vi "log analysis_gps.vi"() -> ()   [LabVIEW 2019] (continued)
178.674099\t119.545505\t7.850800\t-0.685777\t0.071314\t-179.533156\t0.281000\t0.057000\n\t\n15:42:58.0\tlog_raw\tgps_raw\t\tsystem status\tnormal 2 27.600000 0 0\trobot status\t178.530847\t119.555487\t7.852900\t-0.681543\t0.074991\t-178.454031\t0.250000\t0.099000\n\t\n15:42:58.5\tlog_raw\tgps_raw\t\tsystem status\tnormal 2 27.700000 0 0\trobot status\t178.388527\t119.563164\t7.854800\t-0.589771\t-0.039623\t-177.691683\t0.355000\t-0.076000\n\t\n15:42:59.0\tlog_raw\tgps_raw\t#INSPVAXA,USB3,0,48.0,FINESTEERING,2107,283397.000,02008000,471d,15824;INS_ALIGNMENT_COMPLETE,INS_RTKFIXED,37.37120756158,126.72284723555,7.8555,22.3000,0.0154,-0.2918,-0.0108,-0.634674297,-0.085063668,267.337636421,0.4417,0.2975,0.5723,0.1133,0.0929,0.0782,0.0967,0.1016,4.9878,0f000001,0*8fe1902c\n\tsystem status\tnormal 2 27.800000 0 0\trobot status\t178.231220\t119.569034\t7.855500\t-0.634674\t-0.085064\t-177.337636\t0.230000\t0.096000\n\t\n15:42:59.5\tlog_raw\tgps_raw\t\tsystem status\tnormal 2 27.900000 0 0\trobot status\t178.104677\t119.573703\t7.856600\t-0.691004\t0.066213\t-177.257686\t0.292000\t-0.004000\n\t\n15:43:00.0\tlog_raw\tgps_raw\t\tsystem status\tnormal 2 27.800000 0 0\trobot status\t178.014430\t119.582125\t7.857700\t-0.560476\t0.164777\t-177.081673\t0.289000\t-0.046000\n\t\n15:43:00.5\tlog_raw\tgps_raw\t#INSPVAXA,USB3,0,46.0,FINESTEERING,2107,283398.500,02000000,471d,15824;INS_ALIGNMENT_COMPLETE,INS_RTKFIXED,37.37120769045,126.72284269521,7.8578,22.3000,0.0082,-0.2767,-0.0005,-0.866355787,-0.085585905,267.490403578,0.4423,0.2980,0.5726,0.1137,0.0929,0.0782,0.0966,0.1016,4.9900,0f000001,0*ee0dcbd5\n\tsystem status\tnormal 2 27.900000 0 0\trobot status\t177.829044\t119.583345\t7.857800\t-0.866356\t-0.085586\t-177.490404\t0.291000\t-0.016000\n\t\n15:43:01.0\tlog_raw\tgps_raw\t#INSPVAXA,USB3,0,46.0,FINESTEERING,2107,283399.000,02000000,471d,15824;INS_ALIGNMENT_COMPLETE,INS_RTKFIXED,37.37120774226,126.72284145946,7.8578,22.3000,0.0199,-0.3107,0.0000,-0.861107937,-0.016080151,267.485200406,0.4423,0.2980,0.5726,0.1137,0.0929,0.0782,0.0966,0.1016,4.9900,0f000001,0*0e2ee5eb\n\tsystem status\tnormal 2 27.900000 0 0\trobot status\t177.719583\t119.589098\t7.857800\t-0.861108\t-0.016080\t-177.485200\t0.296000\t-0.009000\n\t\n15:43:01.5\tlog_raw\tgps_raw\t\tsystem status\tnormal 2 27.900000 0 0\trobot status\t177.583399\t119.592846\t7.858100\t-0.914716\t-0.066763\t-177.678459\t0.294000\t-0.080000\n\t\n15:43:02.0\tlog_raw\tgps_raw\t\tsystem status\tnormal 2 27.900000 0 0\trobot status\t177.430654\t119.597965\t7.857300\t-1.000637\t-0.107557\t-178.105388\t0.316000\t-0.089000\n\t\n15:43:02.5\tlog_raw\tgps_raw\t#INSPVAXA,USB3,0,49.0,FINESTEERING,2107,283400.500,02008000,471d,15824;INS_ALIGNMENT_COMPLETE,INS_RTKFIXED,37.37120790493,126.72283644279,7.8568,22.3000,0.0415,-0.3200,-0.0102,-0.992860449,-0.204263174,269.501464610,0.4444,0.2986,0.5733,0.1141,0.0930,0.0783,0.0966,0.1016,4.9910,0f000001,0*94df5475\n\tsystem status\tnormal 2 27.600000 0 0\trobot status\t177.275215\t119.607161\t7.856800\t-0.992860\t-0.204263\t-179.501465\t0.300000\t-0.089000\n\t\n15:43:03.0\tlog_raw\tgps_raw\t\tsystem status\tnormal 2 27.400000 0 0\trobot status\t177.149847\t119.619751\t7.856100\t-1.032172\t-0.114714\t178.589566\t0.300000\t-0.076000\n\t\n15:43:03.5\tlog_raw\tgps_raw\t#INSPVAXA,USB3,0,51.0,FINESTEERING,2107,283401.500,02008000,471d,15824;INS_ALIGNMENT_COMPLETE,INS_RTKFIXED,37.37120822785,126.72283327218,7.8567,22.3000,0.0378,-0.2848,0.0013,-0.896017543,0.041472970,274.456577076,0.4448,0.2985,0.5735,0.1139,0.0930,0.0783,0.0966,0.1016,4.9907,0f000001,0*a1fc700f\n\tsystem status\tnormal 2 27.300000 4 0\trobot status\t177.008302\t119.641208\t7.856600\t-0.892681\t-0.081437\t175.816173\t0.307000\t-0.101000\n\t\n15:43:04.0\tlog_raw\tgps_raw\t#INSPVAXA,USB3,0,51.0,FINESTEERING,2107,283402.000,02008000,471d,15824;INS_ALIGNMENT_COMPLETE,INS_RTKFIXED,37.37120847864,126.72283165681,7.8567,22.3000,0.0753,-0.3061,0.0004,-0.849514538,-0.111394273,277.112069112,0.4448,0.2985,0.5735,0.1139,0.0930,0.0783,0.0966,0.1016,4.9907,0f000001,0*e592cbf0\n\tsystem status\tnormal 2 27.200000 4 0\trobot status\t176.851281\t119.670843\t7.856700\t-0.849515\t-0.111394\t172.887931\t0.290000\t-0.092000\n\t\n15:43:04.5\tlog_raw\tgps_raw\t#INSPVAXA,USB3,0,40.0,FINESTEERING,2107,283402.500,02008000,471d,15824;INS_ALIGNMENT_COMPLETE,INS_RTKFIXED,37.37120871914,126.72283047198,7.8552,22.3000,0.0392,-0.0732,-0.0063,-0.879415981,-0.139080353,278.991486756,0.4452,0.2985,0.5736,0.1139,0.0932,0.0783,0.0967,0.1016,4.9892,0f000001,0*49d1c048\n\tsystem status\tnormal 2 27.500000 0 0\trobot status\t176.746330\t119.697537\t7.855200\t-0.879416\t-0.139080\t171.008513\t0.083000\t-0.016000\n\t\n15:43:05.0\tlog_raw\tgps_raw\t#INSPVAXA,USB3,0,40.0,FINESTEERING,2107,283403.000,02008000,471d,15824;INS_ALIGNMENT_COMPLETE,INS_RTKFIXED,37.37120908297,126.72282892192,7.8525,22.3000,0.0902,-0.2460,-0.0094,-0.757562601,-0.250041594,280.800208389,0.4452,0.2985,0.5736,0.1139,0.0932,0.0783,0.0967,0.1016,4.9892,0f000001,0*49bd1315\n\tsystem status\tnormal 2 27.600000 0 0\trobot status\t176.609029\t119.737920\t7.852500\t-0.757563\t-0.250042\t169.199792\t0.253000\t-0.048000\n\t\n15:43:05.5\tlog_raw\tgps_raw\t#INSPVAXA,USB3,0,49.5,FINESTEERING,2107,283403.500,02008000,471d,15824;INS_ALIGNMENT_COMPLETE,INS_RTKFIXED,37.37120946303,126.72282732667,7.8498,22.3000,0.0944,-0.2806,-0.0193,-0.668842152,-0.504747549,282.253589377,0.4448,0.2984,0.5737,0.1136,0.0933,0.0783,0.0967,0.1016,4.9866,0f000001,0*5936c3a3\n\tsystem status\tnormal 2 27.600000 0 0\trobot status\t176.467724\t119.780103\t7.849800\t-0.668842\t-0.504748\t167.746411\t0.286000\t-0.039000\n\t\n15:43:06.0\tlog_raw\tgps_raw\t\tsystem status\tnormal 2 27.700000 0 0\trobot status\t176.338393\t119.821680\t7.846400\t-0.619203\t-0.637590\t166.743344\t0.300000\t-0.021000\n\t\n15:43:06.5\tlog_raw\tgps_raw\t#INSPVAXA,USB3,0,44.5,FINESTEERING,2107,283404.500,02000000,471d,15824;INS_ALIGNMENT_COMPLETE,INS_RTKFIXED,37.37121031708,126.72282412618,7.8426,22.3000,0.0922,-0.2745,-0.0175,-0.508504474,-0.605332941,283.953665433,0.4448,0.2984,0.5737,0.1137,0.0932,0.0783,0.0967,0.1016,4.9838,0f000001,0*f5451d9e\n\tsystem status\tnormal 2 27.800000 0 0\trobot status\t176.184230\t119.874896\t7.842600\t-0.508504\t-0.605333\t166.046335\t0.306000\t0.002000\n\t\n15:43:07.0\tlog_raw\tgps_raw\t\tsystem status\tnormal 2 27.800000 0 0\trobot status\t176.058492\t119.920630\t7.837600\t-0.353083\t-0.545601\t165.722125\t0.254000\t-0.062000\n\t\n15:43:07.5\tlog_raw\tgps_raw\t#INSPVAXA,USB3,0,43.5,FINESTEERING,2107,283405.500,02000000,471d,15824;INS_ALIGNMENT_COMPLETE,INS_RTKFIXED,37.37121122876,126.72282101701,7.8318,22.3000,0.1002,-0.2755,-0.0247,-0.139047561,-0.305791959,284.480251115,0.4442,0.2983,0.5736,0.1136,0.0932,0.0782,0.0967,0.1016,4.9810,0f000001,0*98e81a7f\n\tsystem status\tnormal 2 27.900000 0 0\trobot status\t175.908825\t119.976084\t7.831800\t-0.139048\t-0.305792\t165.519749\t0.289000\t-0.013000\n\t\n15:43:08.0\tlog_raw\tgps_raw\t#INSPVAXA,USB3,0,43.5,FINESTEERING,2107,283406.000,02000000,471d,15824;INS_ALIGNMENT_COMPLETE,INS_RTKFIXED,37.37121169397,126.72281951047,7.8268,22.3000,0.1108,-0.2868,-0.0208,0.099651120,-0.291418852,284.605342241,0.4442,0.2983,0.5736,0.1136,0.0932,0.0782,0.0967,0.1016,4.9810,0f000001,0*55374de0\n\tsystem status\tnormal 2 27.900000 0 0\trobot status\t175.775378\t120.027718\t7.826800\t0.099651\t-0.291419\t165.394658\t0.302000\t0.023000\n\t\n15:43:08.5\tlog_raw\tgps_raw\t#INSPVAXA,USB3,0,49.5,FINESTEERING,2107,283406.500,02000000,471d,15824;INS_ALIGNMENT_COMPLETE,INS_RTKFIXED,37.37121212971,126.72281808061,7.8238,22.3000,0.1054,-0.2584,-0.0109,0.137601109,-0.336757445,284.673154927,0.4438,0.2982,0.5735,0.1136,0.0935,0.0782,0.0967,0.1016,4.9790,0f000001,0*e60377c5\n\tsystem status\tnormal 2 27.900000 0 0\trobot status\t175.648723\t120.076081\t7.823800\t0.137601\t-0.336757\t165.326845\t0.291000\t0.030000\n\t\n15:43:09.0\tlog_raw\tgps_raw\t#INSPVAXA,USB3,0,49.5,FINESTEERING,2107,283407.000,02000000,471d,15824;INS_ALIGNMENT_COMPLETE,INS_RTKFIXED,37.37121262713,126.72281640166,7.8194,22.3000,0.1069,-0.3011,-0.0264,0.109820957,-0.453228449,284.767303943,0.4438,0.2982,0.5735,0.1136,0.0935,0.0782,0.0967,0.1016,4.9790,0f000001,0*3f427643\n\tsystem status\tnormal 2 27.900000 0 0\trobot status\t175.500005\t120.131290\t7.819400\t0.109821\t-0.453228\t165.232696\t0.243000\t0.059000\n\t\n15:43:09.5\tlog_raw\tgps_raw\t#INSPVAXA,USB3,0,48.0,FINESTEERING,2107,283407.500,02000000,471d,15824;INS_ALIGNMENT_COMPLETE,INS_RTKFIXED,37.37121306195,126.72281499649,7.8146,22.3000,0.1240,-0.3347,-0.0132,0.207501666,-0.436324558,284.580204536,0.4442,0.2982,0.5735,0.1137,0.0934,0.0782,0.0967,0.1017,4.9771,0f000001,0*8c70faff\n\tsystem status\tnormal 2 27.800000 0 0\trobot status\t175.375537\t120.179551\t7.814600\t0.207502\t-0.436325\t165.419795\t0.329000\t0.008000\n\t\n15:43:10.0\tlog_raw\tgps_raw\t#INSPVAXA,USB3,0,48.0,FINESTEERING,2107,283408.000,02000000,471d,15824;INS_ALIGNMENT_COMPLETE,INS_RTKFIXED,37.37121354821,126.72281341269,7.8101,22.3000,0.1116,-0.3074,-0.0226,0.525843943,-0.411708262,284.163389107,0.4442,0.2982,0.5735,0.1137,0.0934,0.0782,0.0967,0.1017,4.9771,0f000001,0*c1d0c0d0\n\tsystem status\tnormal 2 27.800000 0 0\trobot status\t175.235246\t120.233521\t7.810100\t0.525844\t-0.411708\t165.836611\t0.230000\t0.127000\n\t\n15:43:10.5\tlog_raw\tgps_raw\t#INSPVAXA,USB3,0,44.0,FINESTEERING,2107,283408.500,02000000,471d,15824;INS_ALIGNMENT_COMPLETE,INS_RTKFIXED,37.37121398943,126.72281189680,7.8055,22.3000,0.1138,-0.2746,-0.0275,0.675393790,-0.337920064,283.271814178,0.4441,0.2981,0.5734,0.1138,0.0936,0.0782,0.0967,0.1017,4.9759,0f000001,0*ad4dbf0b\n\tsystem status\tnormal 2 27.700000 0 0\trobot status\t175.100971\t120.282493\t7.805500\t0.675394\t-0.337920\t166.728186\t0.325000\t-0.019000\n\t\n15:43:11.0\tlog_raw\tgps_raw\t#INSPVAXA,USB3,0,44.0,FINESTEERING,2107,283409.000,02000000,471d,15824;INS_ALIGNMENT_COMPLETE,INS_RTKFIXED,37.37121442754,126.72281035382,7.7998,22.3000,0.1067,-0.2915,-0.0280,0.822552391,-0.280575690,282.018938014,0.4441,0.2981,0.5734,0.1138,0.0936,0.0782,0.0967,0.1017,4.9759,0f000001,0*67fc65b3\n\tsystem status\tnormal 2 27.500000 0 0\trobot status\t174.964297\t120.331119\t7.799800\t0.822552\t-0.280576\t167.981062\t0.275000\t0.073000\n\t\n15:43:11.5\tlog_raw\tgps_raw\t#INSPVAXA,USB3,0,49.0,FINESTEERING,2107,283409.500,02000000,471d,15824;INS_ALIGNMENT_COMPLETE,INS_RTKFIXED,37.37121478666,126.72280882264,7.7967,22.3000,0.1036,-0.2896,-0.0167,0.817605955,-0.233379824,280.341751622,0.4442,0.2981,0.5733,0.1139,0.0934,0.0782,0.0968,0.1017,4.9750,0f000001,0*d948c100\n\tsystem status\tnormal 2 27.300000 0 0\trobot status\t174.828667\t120.370979\t7.796700\t0.817606\t-0.233380\t169.658248\t0.311000\t0.063000\n\t\n15:43:12.0\tlog_raw\tgps_raw\t#INSPVAXA,USB3,0,49.0,FINESTEERING,2107,283410.000,02000000,471d,15824;INS_ALIGNMENT_COMPLETE,INS_RTKFIXED,37.37121511578,126.72280728000,7.7945,22.3000,0.0801,-0.2984,-0.0279,0.678250969,-0.053144715,278.846138365,0.4442,0.2981,0.5733,0.1139,0.0934,0.0782,0.0968,0.1017,4.9750,0f000001,0*ea5c4675\n\tsystem status\tnormal 2 27.400000 0 0\trobot status\t174.692023\t120.407509\t7.794500\t0.678251\t-0.053145\t171.153862\t0.300000\t0.053000\n\t\n15:43:12.5\tlog_raw\tgps_raw\t#INSPVAXA,USB3,0,50.0,FINESTEERING,2107,283410.500,02000000,471d,15824;INS_ALIGNMENT_COMPLETE,INS_RTKFIXED,37.37121543638,126.72280574107,7.7946,22.3000,0.0881,-0.2945,-0.0308,0.799531851,-0.090684476,277.306863329,0.4440,0.2981,0.5734,0.1139,0.0931,0.0782,0.0968,0.1016,4.9749,0f000001,0*8afda85b\n\tsystem status\tnormal 2 27.400000 0 0\trobot status\t174.555707\t120.443093\t7.794600\t0.799532\t-0.090684\t172.693137\t0.303000\t0.051000\n\t\n15:43:13.0\tlog_raw\tgps_raw\t#INSPVAXA,USB3,0,50.0,FINESTEERING,2107,283411.000,02000000,471d,15824;INS_ALIGNMENT_COMPLETE,INS_RTKFIXED,37.37121573081,126.72280419949,7.7932,22.3000,0.0856,-0.2853,-0.0213,0.874963838,0.088876900,275.787048290,0.4440,0.2981,0.5734,0.1139,0.0931,0.0782,0.0968,0.1016,4.9749,0f000001,0*8eff61ca\n\tsystem status\tnormal 2 27.400000 0 0\trobot status\t174.419156\t120.475773\t7.793200\t0.874964\t0.088877\t174.212952\t0.295000\t0.043000\n\t\n15:43:13.5\tlog_raw\tgps_raw\t#INSPVAXA,USB3,0,47.0,FINESTEERING,2107,283411.500,02000000,471d,15824;INS_ALIGNMENT_COMPLETE,INS_RTKFIXED,37.37121596120,126.72280262366,7.7899,22.3000,0.0704,-0.2845,-0.0255,0.751254674,0.247689552,274.576260626,0.4438,0.2979,0.5732,0.1139,0.0930,0.0782,0.0968,0.1016,4.9755,0f000001,0*e84a82b6\n\tsystem status\tnormal 2 27.600000 0 0\trobot status\t174.279572\t120.501346\t7.789900\t0.751255\t0.247690\t175.423739\t0.301000\t0.040000\n\t\n15:43:14.0\tlog_raw\tgps_raw\t#INSPVAXA,USB3,0,47.0,FINESTEERING,2107,283412.000,02000000,471d,15824;INS_ALIGNMENT_COMPLETE,INS_RTKFIXED,37.37121617740,126.72280126848,7.7873,22.3000,0.0873,-0.4025,-0.0234,0.616180414,0.315751061,274.011690427,0.4438,0.2979,0.5732,0.1139,0.0930,0.0782,0.0968,0.1016,4.9755,0f000001,0*aa33c281\n\tsystem status\tnormal 2 27.600000 0 0\trobot status\t174.159532\t120.525343\t7.787300\t0.616180\t0.315751\t175.988310\t0.464000\t-0.135000\n\t\n15:43:14.5\tlog_raw\tgps_raw\t#INSPVAXA,USB3,0,49.0,FINESTEERING,2107,283412.500,02000000,471d,15824;INS_ALIGNMENT_COMPLETE,INS_RTKFIXED,37.37121638911,126.72279968745,7.7862,22.3000,0.0846,-0.3281,-0.0274,0.679733503,0.333649216,273.348704844,0.4441,0.2978,0.5733,0.1135,0.0929,0.0782,0.0967,0.1016,4.9761,0f000001,0*b2c3b0d0\n\tsystem status\tnormal 2 27.700000 0 0\trobot status\t174.019487\t120.548843\t7.786200\t0.679734\t0.333649\t176.651295\t0.285000\t0.061000\n\t\n15:43:15.0\tlog_raw\tgps_raw\t#INSPVAXA,USB3,0,49.0,FINESTEERING,2107,283413.000,02000000,471d,15824;INS_ALIGNMENT_COMPLETE,INS_RTKFIXED,37.37121660586,126.72279809431,7.7843,22.3000,0.0703,-0.2977,-0.0214,0.740409973,0.249491929,272.781944471,0.4441,0.2978,0.5733,0.1135,0.0929,0.0782,0.0967,0.1016,4.9761,0f000001,0*f60b4ece\n\tsystem status\tnormal 2 27.700000 0 0\trobot status\t173.878369\t120.572902\t7.784300\t0.740410\t0.249492\t177.218056\t0.285000\t0.039000\n\t\n15:43:15.5\tlog_raw\tgps_raw\t#INSPVAXA,USB3,0,52.0,FINESTEERING,2107,283413.500,02000000,471d,15824;INS_ALIGNMENT_COMPLETE,INS_RTKFIXED,37.37121678011,126.72279647899,7.7842,22.3000,0.0611,-0.2896,-0.0156,0.541768048,0.276425000,272.440789392,0.4443,0.2978,0.5734,0.1137,0.0930,0.0783,0.0967,0.1016,4.9772,0f000001,0*dee707a2\n\tsystem status\tnormal 2 27.800000 0 0\trobot status\t173.735287\t120.592244\t7.784200\t0.541768\t0.276425\t177.559211\t0.303000\t0.023000\n\t\n15:43:16.0\tlog_raw\tgps_raw\t#INSPVAXA,USB3,0,52.0,FINESTEERING,2107,283414.000,02000000,471d,15824;INS_ALIGNMENT_COMPLETE,INS_RTKFIXED,37.37121695844,126.72279487453,7.7833,22.3000,0.0562,-0.2987,-0.0221,0.305746211,0.346254228,272.319331007,0.4443,0.2978,0.5734,0.1137,0.0930,0.0783,0.0967,0.1016,4.9772,0f000001,0*5e10dc17\n\tsystem status\tnormal 2 27.800000 0 0\trobot status\t173.593167\t120.612039\t7.783300\t0.305746\t0.346254\t177.680669\t0.255000\t0.072000\n\t\n15:43:16.5\tlog_raw\tgps_raw\t#INSPVAXA,USB3,0,50.0,FINESTEERING,2107,283414.500,02000000,471d,15824;INS_ALIGNMENT_COMPLETE,INS_RTKFIXED,37.37121711379,126.72279330042,7.7828,22.3000,0.0616,-0.3002,-0.0329,0.276756604,0.384134091,272.213822291,0.4446,0.2977,0.5735,0.1137,0.0931,0.0783,0.0967,0.1016,4.9781,0f000001,0*58d30e64\n\tsystem status\tnormal 2 27.800000 0 0\trobot status\t173.453735\t120.629283\t7.782800\t0.276757\t0.384134\t177.786178\t0.325000\t-0.049000\n\t\n15:43:17.0\tlog_raw\tgps_raw\t#INSPVAXA,USB3,0,50.0,FINESTEERING,2107,283415.000,02000000,471d,15824;INS_ALIGNMENT_COMPLETE,INS_RTKFIXED,37.37121729157,126.72279172002,7.7811,22.3000,0.0636,-0.2842,-0.0222,0.415011946,0.501817180,272.226800833,0.4446,0.2977,0.5735,0.1137,0.0931,0.0783,0.0967,0.1016,4.9781,0f000001,0*6d269faa\n\tsystem status\tnormal 2 27.900000 0 0\trobot status\t173.313745\t120.649017\t7.781100\t0.415012\t0.501817\t177.773199\t0.252000\t0.068000\n\t\n15:43:17.5\tlog_raw\tgps_raw\t#INSPVAXA,USB3,0,47.5,FINESTEERING,2107,283415.500,02000000,471d,15824;INS_ALIGNMENT_COMPLETE,INS_RTKFIXED,37.37121745091,126.72279017522,7.7808,22.3000,0.0665,-0.2955,-0.0219,0.380400509,0.552941969,272.302095056,0.4463,0.2979,0.5741,0.1141,0.0931,0.0783,0.0967,0.1016,4.9784,0f000001,0*a1df6ecd\n\tsystem status\tnormal 2 27.900000 0 0\trobot status\t173.176909\t120.666704\t7.780800\t0.380401\t0.552942\t177.697905\t0.302000\t-0.016000\n\t\n15:43:18.0\tlog_raw\tgps_raw\t#INSPVAXA,USB3,0,47.5,FINESTEERING,2107,283416.000,02000000,471d,15824;INS_ALIGNMENT_COMPLETE,INS_RTKFIXED,37.37121761561,126.72278863452,7.7803,22.3000,0.0694,-0.2870,-0.0195,0.176632637,0.631844769,272.368772552,0.4463,0.2979,0.5741,0.1141,0.0931,0.0783,0.0967,0.1016,4.9784,0f000001,0*101cc811\n\tsystem status\tnormal 2 27.900000 0 0\trobot status\t173.040437\t120.684986\t7.780300\t0.176633\t0.631845\t177.631227\t0.294000\t-0.025000\n\t\n15:43:18.5\tlog_raw\tgps_raw\t#INSPVAXA,USB3,0,48.5,FINESTEERING,2107,283416.500,02000000,471d,15824;INS_ALIGNMENT_COMPLETE,INS_RTKFIXED,37.37121775832,126.72278713599,7.7826,22.3000,0.0697,-0.2192,-0.0178,0.097264946,0.637535268,272.514997324,0.4476,0.2980,0.5744,0.1141,0.0933,0.0783,0.0967,0.1016,4.9780,0f000001,0*de8fa7bd\n\tsystem status\tnormal 2 27.900000 0 0\trobot status\t172.907699\t120.700827\t7.782600\t0.097265\t0.637535\t177.485003\t0.270000\t-0.019000\n\t\n15:43:19.0\tlog_raw\tgps_raw\t#INSPVAXA,USB3,0,48.5,FINESTEERING,2107,283417.000,02000000,471d,15824;INS_ALIGNMENT_COMPLETE,INS_RTKFIXED,37.37121791673,126.72278556304,7.7837,22.3000,0.0663,-0.3100,-0.0205,0.059332705,0.713618061,272.644367778,0.4476,0.2980,0.5744,0.1141,0.0933,0.0783,0.0967,0.1016,4.9780,0f000001,0*0eada2f0\n\tsystem status\tnormal 2 27.900000 0 0\trobot status\t172.768370\t120.718411\t7.783700\t0.059333\t0.713618\t177.355632\t0.311000\t-0.019000\n\t\n15:43:19.5\tlog_raw\tgps_raw\t#INSPVAXA,USB3,0,49.5,FINESTEERING,2107,283417.500,02000000,471d,15824;INS_ALIGNMENT_COMPLETE,INS_RTKFIXED,37.37121805927,126.72278401761,7.7854,22.3000,0.0733,-0.3034,-0.0199,-0.089736281,0.682506792,272.907308438,0.4484,0.2980,0.5747,0.1140,0.0932,0.0783,0.0967,0.1016,4.9768,0f000001,0*d6901b99\n\tsystem status\tnormal 2 27.900000 0 0\trobot status\t172.631478\t120.734234\t7.785400\t-0.089736\t0.682507\t177.092692\t0.296000\t-0.026000\n\t\n15:43:20.0\tlog_raw\tgps_raw\t#INSPVAXA,USB3,0,49.5,FINESTEERING,2107,283418.000,02000000,471d,15824;INS_ALIGNMENT_COMPLETE,INS_RTKFIXED,37.37121822786,126.72278229435,7.7864,22.3000,0.0757,-0.2957,-0.0211,-0.132925530,0.544261576,273.127275115,0.4484,0.2980,0.5747,0.1140,0.0932,0.0783,0.0967,0.1016,4.9768,0f000001,0*048d27a0\n\tsystem status\tnormal 2 27.900000 0 0\trobot status\t172.478835\t120.752948\t7.786400\t-0.132926\t0.544262\t176.872725\t0.297000\t-0.022000\n\t\n15:43:20.5\tlog_raw\tgps_raw\t#INSPVAXA,USB3,0,48.5,FINESTEERING,2107,283418.500,02000000,471d,15824;INS_ALIGNMENT_COMPLETE,INS_RTKFIXED,37.37121838802,126.72278063938,7.7901,22.3000,0.0744,-0.3140,-0.0189,-0.074171217,0.383892357,273.451467378,0.4479,0.2973,0.5742,0.1138,0.0931,0.0783,0.0966,0.1015,4.9755,0f000001,0*a7f0c313\n\tsystem status\tnormal 2 27.900000 0 0\trobot status\t172.332240\t120.770726\t7.790100\t-0.074171\t0.383892\t176.548533\t0.318000\t-0.017000\n\t\n15:43:21.0\tlog_raw\tgps_raw\t#INSPVAXA,USB3,0,48.5,FINESTEERING,2107,283419.000,02000000,471d,15824;INS_ALIGNMENT_COMPLETE,INS_RTKFIXED,37.37121856246,126.72277896327,7.7932,22.3000,0.0727,-0.3040,-0.0212,-0.024906260,0.224477115,273.793356519,0.4479,0.2973,0.5742,0.1138,0.0931,0.0783,0.0966,0.1015,4.9755,0f000001,0*a3bde9c9\n\tsystem status\tnormal 2 27.900000 0 0\trobot status\t172.183773\t120.790089\t7.793200\t-0.024906\t0.224477\t176.206643\t0.309000\t-0.022000\n\t\n15:43:21.5\tlog_raw\tgps_raw\t#INSPVAXA,USB3,0,48.5,FINESTEERING,2107,283419.500,02000000,471d,15824;INS_ALIGNMENT_COMPLETE,INS_RTKFIXED,37.37121873521,126.72277734418,7.7960,22.3000,0.0758,-0.3154,-0.0078,-0.021214683,0.148956013,274.268869002,0.4473,0.2969,0.5737,0.1137,0.0929,0.0783,0.0966,0.1015,4.9747,0f000001,0*df94383f\n\tsystem status\tnormal 2 27.800000 0 0\trobot status\t172.040357\t120.809265\t7.796000\t-0.021215\t0.148956\t175.731131\t0.302000\t-0.030000\n\t\n15:43:22.0\tlog_raw\tgps_raw\t#INSPVAXA,USB3,0,48.5,FINESTEERING,2107,283420.000,02000000,471d,15824;INS_ALIGNMENT_COMPLETE,INS_RTKFIXED,37.37121893456,126.72277571347,7.7975,22.3000,0.0783,-0.3033,-0.0206,0.031637504,0.132212699,274.926400235,0.4473,0.2969,0.5737,0.1137,0.0929,0.0783,0.0966,0.1015,4.9747,0f000001,0*9f2f7546\n\tsystem status\tnormal 2 27.800000 0 0\trobot status\t171.895911\t120.831393\t7.797500\t0.031638\t0.132213\t175.073600\t0.292000\t-0.032000\n\t\n15:43:22.5\tlog_raw\tgps_raw\t#DUALANTENNAHEADINGA,USB3,0,49.5,FINESTEERING,2107,283420.500,02000000,d426,15824;SOL_COMPUTED,L1_FLOAT,-1.000000000,234.407104492,43.477504730,0.0,94.985305786,98.100028992,\"631T\",12,5,5,4,04,00,20,03*0ae8aff3\n\tsystem status\tnormal 2 27.700000 0 0\trobot status\t171.753456\t120.854339\t7.798900\t-0.085196\t0.035882\t174.255991\t0.221000\t-0.159000\n\t\n15:43:23.0\tlog_raw\tgps_raw\t#INSPVAXA,USB3,0,49.5,FINESTEERING,2107,283421.000,02000000,471d,15824;INS_ALIGNMENT_COMPLETE,INS_RTKFIXED,37.37121936373,126.72277250548,7.7996,22.3000,0.0650,-0.2575,-0.0195,-0.339414237,-0.334723379,276.547401542,0.4463,0.2965,0.5732,0.1137,0.0928,0.0782,0.0966,0.1015,4.9752,0f000001,0*ec1dc2f2\n\tsystem status\tnormal 2 27.800000 0 0\trobot status\t171.611753\t120.879030\t7.799600\t-0.339414\t-0.334723\t173.452598\t0.209000\t-0.063000\n\t\n15:43:23.5\tlog_raw\tgps_raw\t#INSPVAXA,USB3,0,51.5,FINESTEERING,2107,283421.500,02000000,471d,15824;INS_ALIGNMENT_COMPLETE,INS_RTKFIXED,37.37121958674,126.72277110428,7.8012,22.3000,0.0748,-0.3049,-0.0167,-0.332988455,-0.342081628,277.184622547,0.4456,0.2963,0.5729,0.1138,0.0929,0.0782,0.0966,0.1015,4.9763,0f000001,0*dbd926c2\n\tsystem status\tnormal 2 27.800000 0 0\trobot status\t171.487637\t120.903783\t7.801200\t-0.332988\t-0.342082\t172.815377\t0.318000\t-0.101000\n\t\n15:43:24.0\tlog_raw\tgps_raw\t#INSPVAXA,USB3,0,51.5,FINESTEERING,2107,283422.000,02000000,471d,15824;INS_ALIGNMENT_COMPLETE,INS_RTKFIXED,37.37121986544,126.72276955202,7.8030,22.3000,0.0826,-0.2892,-0.0063,-0.059772273,-0.284356871,277.924098643,0.4456,0.2963,0.5729,0.1138,0.0929,0.0782,0.0966,0.1015,4.9763,0f000001,0*9e39ca32\n\tsystem status\tnormal 2 27.800000 0 0\trobot status\t171.350140\t120.934717\t7.803000\t-0.059772\t-0.284357\t172.075901\t0.355000\t0.036000\n\t\n15:43:24.5\tlog_raw\tgps_raw\t#INSPVAXA,USB3,0,50.0,FINESTEERING,2107,283422.500,02000000,471d,15824;INS_ALIGNMENT_COMPLETE,INS_RTKFIXED,37.37122013933,126.72276801753,7.8064,22.3000,0.0862,-0.2930,-0.0083,0.046604399,-0.149550594,278.523812878,0.4449,0.2961,0.5725,0.1140,0.0927,0.0782,0.0966,0.1015,4.9774,0f000001,0*ad33b229\n\tsystem status\tnormal 2 27.800000 0 0\trobot status\t171.214218\t120.965118\t7.806400\t0.046604\t-0.149551\t171.476187\t0.356000\t0.058000\n\t\n15:43:25.0\tlog_raw\tgps_raw\t#DUALANTENNAHEADINGA,USB3,0,50.0,FINESTEERING,2107,283423.000,02000000,d426,15824;INSUFFICIENT_OBS,NONE,-1.000000000,0.000000000,0.000000000,0.0,0.000000000,0.000000000,\"631T\",14,4,4,3,04,00,20,03*0f5fdb5e\n\tsystem status\tnormal 2 27.800000 0 0\trobot status\t171.078046\t120.996756\t7.808400\t-0.005494\t0.123460\t170.832840\t0.259000\t-0.080000\n\t\n15:43:25.5\tlog_raw\tgps_raw\t#DUALANTENNAHEADINGA,USB3,0,47.0,FINESTEERING,2107,283423.500,02000000,d426,15824;INSUFFICIENT_OBS,NONE,-1.000000000,0.000000000,0.000000000,0.0,0.000000000,0.000000000,\"631T\",14,4,4,3,04,00,20,03*ef3cce1d\n\tsystem status\tnormal 2 27.800000 0 0\trobot status\t170.938637\t121.031056\t7.812000\t0.034428\t0.261804\t170.416684\t0.336000\t0.071000\n\t\n15:43:26.0\tlog_raw\tgps_raw\t#DUALANTENNAHEADINGA,USB3,0,47.0,FINESTEERING,2107,283424.000,02000000,d426,15824;INSUFFICIENT_OBS,NONE,-1.000000000,0.000000000,0.000000000,0.0,0.000000000,0.000000000,\"631T\",14,4,4,3,04,00,20,03*e256c70a\n\tsystem status\tnormal 2 27.900000 0 0\trobot status\t170.798403\t121.067983\t7.814600\t0.069675\t0.182873\t170.117150\t0.288000\t-0.021000\n\t\n15:43:26.5\tlog_raw\tgps_raw\t#INSPVAXA,USB3,0,47.0,FINESTEERING,2107,283424.500,02000000,471d,15824;INS_ALIGNMENT_COMPLETE,INS_RTKFIXED,37.37122139121,126.72276178934,7.8175,22.3000,0.0963,-0.2911,-0.0267,0.160577040,0.027759936,280.115354795,0.4445,0.2959,0.5718,0.1138,0.0927,0.0782,0.0966,0.1015,4.9793,0f000001,0*3cf8e5a0\n\tsystem status\tnormal 2 27.900000 0 0\trobot status\t170.662535\t121.104068\t7.817500\t0.160577\t0.027760\t169.884645\t0.305000\t0.007000\n\t\n15:43:27.0\tlog_raw\tgps_raw\t#INSPVAXA,USB3,0,47.0,FINESTEERING,2107,283425.000,02000000,471d,15824;INS_ALIGNMENT_COMPLETE,INS_RTKFIXED,37.37122172446,126.72276025086,7.8192,22.3000,0.1007,-0.2909,-0.0258,0.166214730,-0.121164674,280.254709896,0.4445,0.2959,0.5718,0.1138,0.0927,0.0782,0.0966,0.1015,4.9793,0f000001,0*7313d272\n\tsystem status\tnormal 2 27.900000 0 0\trobot status\t170.526259\t121.141057\t7.819200\t0.166215\t-0.121165\t169.745290\t0.302000\t0.000000\n\t\n15:43:27.5\tlog_raw\tgps_raw\t#INSPVAXA,USB3,0,49.5,FINESTEERING,2107,283425.500,02000000,471d,15824;INS_ALIGNMENT_COMPLETE,INS_RTKFIXED,37.37122203664,126.72275876247,7.8214,22.3000,0.1014,-0.2752,-0.0310,0.225701911,-0.169314911,280.367326711,0.4448,0.2959,0.5717,0.1139,0.0927,0.0782,0.0966,0.1015,4.9800,0f000001,0*47093191\n\tsystem status\tnormal 2 27.900000 0 0\trobot status\t170.394420\t121.175707\t7.821400\t0.225702\t-0.169315\t169.632673\t0.298000\t0.012000\n\t\n15:43:28.0\tlog_raw\tgps_raw\t#INSPVAXA,USB3,0,49.5,FINESTEERING,2107,283426.000,02000000,471d,15824;INS_ALIGNMENT_COMPLETE,INS_RTKFIXED,37.37122236568,126.72275725314,7.8225,22.3000,0.1015,-0.2829,-0.0297,0.362209359,-0.363441278,280.451922060,0.4448,0.2959,0.5717,0.1139,0.0927,0.0782,0.0966,0.1015,4.9800,0f000001,0*8f1e70f0\n\tsystem status\tnormal 2 27.900000 0 0\trobot status\t170.260726\t121.212228\t7.822500\t0.362209\t-0.363441\t169.548078\t0.300000\t0.013000\n\t\n15:43:28.5\tlog_raw\tgps_raw\t#INSPVAXA,USB3,0,46.5,FINESTEERING,2107,283426.500,02000000,471d,15824;INS_ALIGNMENT_COMPLETE,INS_RTKFIXED,37.37122268854,126.72275568297,7.8242,22.3000,0.1049,-0.3026,-0.0329,0.482516704,-0.388354216,280.500192779,0.4446,0.2958,0.5715,0.1139,0.0928,0.0782,0.0966,0.1016,4.9804,0f000001,0*3c38bbfe\n\tsystem status\tnormal 2 27.900000 0 0\trobot status\t170.121642\t121.248063\t7.824200\t0.482517\t-0.388354\t169.499807\t0.300000\t0.017000\n\t\n15:43:29.0\tlog_raw\tgps_raw\t#INSPVAXA,USB3,0,46.5,FINESTEERING,2107,283427.000,02000000,471d,15824;INS_ALIGNMENT_COMPLETE,INS_RTKFIXED,37.37122302372,126.72275405383,7.8254,22.3000,0.1035,-0.2991,-0.0114,0.517295198,-0.533849099,280.546073073,0.4446,0.2958,0.5715,0.1139,0.0928,0.0782,0.0966,0.1016,4.9804,0f000001,0*317727c1\n\tsystem status\tnormal 2 27.900000 0 0\trobot status\t169.977336\t121.285266\t7.825400\t0.517295\t-0.533849\t169.453927\t0.304000\t0.015000\n\t\n15:43:29.5\tlog_raw\tgps_raw\t#DUALANTENNAHEADINGA,USB3,0,47.5,FINESTEERING,2107,283427.500,02000000,d426,15824;SOL_COMPUTED,L1_FLOAT,-1.000000000,232.849288940,45.452278137,0.0,33.969039917,39.167930603,\"631T\",14,5,5,3,04,00,20,03*a09f33ea\n\tsystem status\tnormal 2 27.900000 0 0\trobot status\t169.836102\t121.320787\t7.826300\t0.302654\t-0.660231\t169.435245\t0.307000\t0.019000\n\t\n15:43:30.0\tlog_raw\tgps_raw\t#INSPVAXA,USB3,0,47.5,FINESTEERING,2107,283428.000,02000000,471d,15824;INS_ALIGNMENT_COMPLETE,INS_RTKFIXED,37.37122367818,126.72275085270,7.8261,22.3000,0.0923,-0.2777,-0.0130,0.140840960,-0.867034330,280.536212812,0.4440,0.2956,0.5711,0.1139,0.0927,0.0781,0.0966,0.1016,4.9804,0f000001,0*209210a7\n\tsystem status\tnormal 2 27.900000 0 0\trobot status\t169.693785\t121.357906\t7.826100\t0.140841\t-0.867034\t169.463787\t0.287000\t0.032000\n\t\n15:43:30.5\tlog_raw\tgps_raw\t#INSPVAXA,USB3,0,48.5,FINESTEERING,2107,283428.500,02000000,471d,15824;INS_ALIGNMENT_COMPLETE,INS_RTKFIXED,37.37122400199,126.72274933790,7.8267,22.3000,0.0859,-0.2878,-0.0061,0.135588255,-0.903172735,280.268648781,0.4433,0.2955,0.5708,0.1138,0.0926,0.0781,0.0967,0.1016,4.9799,0f000001,0*057639e6\n\tsystem status\tnormal 2 27.800000 0 0\trobot status\t169.559607\t121.393847\t7.826700\t0.135588\t-0.903173\t169.731351\t0.321000\t-0.008000\n\t\n15:43:31.0\tlog_raw\tgps_raw\t#INSPVAXA,USB3,0,48.5,FINESTEERING,2107,283429.000,02000000,471d,15824;INS_ALIGNMENT_COMPLETE,INS_RTKFIXED,37.37122433213,126.72274779084,7.8272,22.3000,0.0909,-0.2670,-0.0074,0.199966599,-0.926566199,279.797605539,0.4433,0.2955,0.5708,0.1138,0.0926,0.0781,0.0967,0.1016,4.9799,0f000001,0*cc69b281\n\tsystem status\tnormal 2 27.800000 0 0\trobot status\t169.422570\t121.430490\t7.827200\t0.199967\t-0.926566\t170.202394\t0.313000\t-0.005000\n\t\n15:43:31.5\tlog_raw\tgps_raw\t#DUALANTENNAHEADINGA,USB3,0,47.0,FINESTEERING,2107,283429.500,02000000,d426,15824;SOL_COMPUTED,L1_FLOAT,-1.000000000,232.988739014,45.471614838,0.0,34.093307495,39.104740143,\"631T\",13,5,5,3,04,00,20,03*ea83c899\n\tsystem status\tnormal 2 27.700000 0 0\trobot status\t169.285533\t121.463899\t7.828400\t0.111231\t-0.876345\t170.815505\t0.344000\t-0.032000\n\t\n15:43:32.0\tlog_raw\tgps_raw\t#INSPVAXA,USB3,0,47.0,FINESTEERING,2107,283430.000,02000000,471d,15824;INS_ALIGNMENT_COMPLETE,INS_RTKFIXED,37.37122492622,126.72274472809,7.8296,22.3000,0.0738,-0.2911,-0.0264,0.111413714,-0.624845931,278.508262088,0.4425,0.2951,0.5706,0.1137,0.0926,0.0781,0.0967,0.1016,4.9798,0f000001,0*f0033656\n\tsystem status\tnormal 2 27.700000 0 0\trobot status\t169.151277\t121.496431\t7.829600\t0.111414\t-0.624846\t171.491738\t0.257000\t0.079000\n\t\n15:43:32.5\tlog_raw\tgps_raw\t#DUALANTENNAHEADINGA,USB3,0,47.5,FINESTEERING,2107,283430.500,02000000,d426,15824;SOL_COMPUTED,L1_FLOAT,-1.000000000,232.754241943,45.457447052,0.0,33.170593262,38.334568024,\"631T\",11,5,5,3,04,00,20,03*6c1747a2\n\tsystem status\tnormal 2 27.700000 0 0\trobot status\t169.039660\t121.522411\t7.831200\t0.195201\t-0.418566\t172.256598\t0.206000\t-0.012000\n\t\n15:43:33.0\tlog_raw\tgps_raw\t#DUALANTENNAHEADINGA,USB3,0,47.5,FINESTEERING,2107,283431.000,02000000,d426,15824;INSUFFICIENT_OBS,NONE,-1.000000000,0.000000000,0.000000000,0.0,0.000000000,0.000000000,\"631T\",11,4,4,3,04,00,20,03*770d0ff4\n\tsystem status\tnormal 2 27.700000 0 0\trobot status\t168.900201\t121.549726\t7.832600\t0.207939\t-0.291369\t173.020837\t0.292000\t-0.019000\n\t\n15:43:33.5\tlog_raw\tgps_raw\t#DUALANTENNAHEADINGA,USB3,0,49.5,FINESTEERING,2107,283431.500,02000000,d426,15824;SOL_COMPUTED,L1_FLOAT,-1.000000000,232.641693115,45.342384338,0.0,32.806938171,38.312389374,\"631T\",13,5,5,3,04,00,20,03*517ac67c\n\tsystem status\tnormal 2 27.700000 0 0\trobot status\t168.763129\t121.575125\t7.833200\t0.239052\t-0.168936\t173.746686\t0.315000\t-0.017000\n\t\n15:43:34.0\tlog_raw\tgps_raw\t#DUALANTENNAHEADINGA,USB3,0,49.5,FINESTEERING,2107,283432.000,02000000,d426,15824;INSUFFICIENT_OBS,NONE,-1.000000000,0.000000000,0.000000000,0.0,0.000000000,0.000000000,\"631T\",12,4,4,3,04,00,20,03*741ccc0d\n\tsystem status\tnormal 2 27.700000 0 0\trobot status\t168.627413\t121.599030\t7.832800\t0.230599\t-0.017072\t174.432419\t0.286000\t0.028000\n\t\n15:43:34.5\tlog_raw\tgps_raw\t#INSPVAXA,USB3,0,48.0,FINESTEERING,2107,283432.500,02000000,471d,15824;INS_ALIGNMENT_COMPLETE,INS_RTKFIXED,37.37122604855,126.72273724644,7.8341,22.3000,0.0724,-0.2733,-0.0174,0.238872948,0.019909284,274.995506864,0.4422,0.2946,0.5700,0.1135,0.0926,0.0781,0.0966,0.1017,4.9822,0f000001,0*dc53e99c\n\tsystem status\tnormal 2 27.700000 0 0\trobot status\t168.488565\t121.621005\t7.834100\t0.238873\t0.019909\t175.004493\t0.389000\t-0.124000\n\t\n15:43:35.0\tlog_raw\tgps_raw\t#INSPVAXA,USB3,0,48.0,FINESTEERING,2107,283433.000,02000000,471d,15824;INS_ALIGNMENT_COMPLETE,INS_RTKFIXED,37.37122625472,126.72273566540,7.8365,22.3000,0.0706,-0.2887,-0.0199,0.361762560,0.060019418,274.681599898,0.4422,0.2946,0.5700,0.1135,0.0926,0.0781,0.0966,0.1017,4.9822,0f000001,0*5afbe29f\n\tsystem status\tnormal 2 27.800000 0 0\trobot status\t168.348519\t121.643890\t7.836500\t0.361763\t0.060019\t175.318400\t0.237000\t0.102000\n\t\n15:43:35.5\tlog_raw\tgps_raw\t#DUALANTENNAHEADINGA,USB3,0,49.0,FINESTEERING,2107,283433.500,02000000,d426,15824;SOL_COMPUTED,L1_FLOAT,-1.000000000,232.557586670,45.313392639,0.0,32.878929138,38.560791016,\"631T\",14,5,5,3,04,00,20,03*4c22ef33\n\tsystem status\tnormal 2 27.800000 0 0\trobot status\t168.208796\t121.667470\t7.838500\t0.459873\t0.102483\t175.552149\t0.204000\t0.162000\n\t\n15:43:36.0\tlog_raw\tgps_raw\t#DUALANTENNAHEADINGA,USB3,0,49.0,FINESTEERING,2107,283434.000,02000000,d426,15824;INSUFFICIENT_OBS,NONE,-1.000000000,0.000000000,0.000000000,0.0,0.000000000,0.000000000,\"631T\",14,4,4,3,04,00,20,03*0b1b3d45\n\tsystem status\tnormal 2 27.800000 0 0\trobot status\t168.066366\t121.690759\t7.839500\t0.355022\t0.018069\t175.693945\t0.213000\t0.134000\n\t\n15:43:36.5\tlog_raw\tgps_raw\t#INSPVAXA,USB3,0,48.5,FINESTEERING,2107,283434.500,02000000,471d,15824;INS_ALIGNMENT_COMPLETE,INS_RTKFIXED,37.37122687551,126.72273086568,7.8419,22.3000,0.0628,-0.2805,-0.0066,0.210765696,0.014229914,274.274045253,0.4430,0.2944,0.5697,0.1136,0.0924,0.0781,0.0965,0.1017,4.9839,0f000001,0*24038eec\n\tsystem status\tnormal 2 27.900000 0 0\trobot status\t167.923368\t121.712797\t7.841900\t0.210766\t0.014230\t175.725955\t0.327000\t-0.046000\n\t\n15:43:37.0\tlog_raw\tgps_raw\t#INSPVAXA,USB3,0,48.5,FINESTEERING,2107,283435.000,02000000,471d,15824;INS_ALIGNMENT_COMPLETE,INS_RTKFIXED,37.37122709127,126.72272927206,7.8444,22.3000,0.0603,-0.2575,-0.0160,0.234010855,-0.149082924,274.318323900,0.4430,0.2944,0.5697,0.1136,0.0924,0.0781,0.0965,0.1017,4.9839,0f000001,0*fa8bdd9d\n\tsystem status\tnormal 2 27.900000 0 0\trobot status\t167.782207\t121.736745\t7.844400\t0.234011\t-0.149083\t175.681676\t0.214000\t0.030000\n\t\n15:43:37.5\tlog_raw\tgps_raw\t#DUALANTENNAHEADINGA,USB3,0,47.5,FINESTEERING,2107,283435.500,02000000,d426,15824;SOL_COMPUTED,L1_FLOAT,-1.000000000,232.551986694,45.441768646,0.0,33.077499390,38.478469849,\"631T\",15,5,5,3,04,00,20,03*23c7ad13\n\tsystem status\tnormal 2 27.800000 0 0\trobot status\t167.682626\t121.756000\t7.846800\t0.206987\t-0.111840\t175.820882\t0.321000\t0.019000\n\t\n15:43:38.0\tlog_raw\tgps_raw\t#DUALANTENNAHEADINGA,USB3,0,47.5,FINESTEERING,2107,283436.000,02000000,d426,15824;INSUFFICIENT_OBS,NONE,-1.000000000,0.000000000,0.000000000,0.0,0.000000000,0.000000000,\"631T\",13,4,4,3,04,00,20,03*d9c0114b\n\tsystem status\tnormal 2 27.900000 0 0\trobot status\t167.526384\t121.782651\t7.848100\t0.285608\t-0.249343\t175.631180\t0.302000\t-0.013000\n\t\n15:43:38.5\tlog_raw\tgps_raw\t#INSPVAXA,USB3,0,49.5,FINESTEERING,2107,283436.500,02000000,471d,15824;INS_ALIGNMENT_COMPLETE,INS_RTKFIXED,37.37122770448,126.72272483106,7.8496,22.3000,0.0698,-0.3222,-0.0225,0.214534417,-0.208140841,274.430810047,0.4422,0.2943,0.5696,0.1135,0.0924,0.0781,0.0965,0.1016,4.9853,0f000001,0*0962ac25\n\tsystem status\tnormal 2 27.900000 0 0\trobot status\t167.388831\t121.804810\t7.849600\t0.214534\t-0.208141\t175.569190\t0.309000\t0.000000\n\t\n15:43:39.0\tlog_raw\tgps_raw\t#DUALANTENNAHEADINGA,USB3,0,49.5,FINESTEERING,2107,283437.000,02000000,d426,15824;INSUFFICIENT_OBS,NONE,-1.000000000,0.000000000,0.000000000,0.0,0.000000000,0.000000000,\"631T\",13,4,4,3,04,00,20,03*a2375da9\n\tsystem status\tnormal 2 27.900000 0 0\trobot status\t167.248180\t121.829136\t7.849900\t0.116470\t-0.230909\t175.489303\t0.294000\t-0.019000\n\t\n15:43:39.5\tlog_raw\tgps_raw\t#DUALANTENNAHEADINGA,USB3,0,48.0,FINESTEERING,2107,283437.500,02000000,d426,15824;SOL_COMPUTED,L1_FLOAT,-1.000000000,232.550857544,45.494079590,0.0,33.819896698,39.214233398,\"631T\",14,5,5,3,04,00,20,02*42d48a39\n\tsystem status\tnormal 2 27.900000 0 0\trobot status\t167.101802\t121.853303\t7.849200\t-0.004965\t-0.343369\t175.370090\t0.303000\t-0.006000\n\t\n15:43:40.0\tlog_raw\tgps_raw\t#INSPVAXA,USB3,0,48.0,FINESTEERING,2107,283438.000,02000000,471d,15824;INS_ALIGNMENT_COMPLETE,INS_RTKFIXED,37.37122838376,126.72272002570,7.8486,22.3000,0.0782,-0.3050,-0.0191,0.083473353,-0.332948382,274.747622714,0.4419,0.2943,0.5694,0.1131,0.0924,0.0781,0.0965,0.1016,4.9857,0f000001,0*6bacac53\n\tsystem status\tnormal 2 27.900000 0 0\trobot status\t166.963180\t121.880208\t7.848600\t0.083473\t-0.332948\t175.252377\t0.308000\t-0.008000\n\t\n15:43:40.5\tlog_raw\tgps_raw\t#DUALANTENNAHEADINGA,USB3,0,49.0,FINESTEERING,2107,283438.500,02000000,d426,15824;SOL_COMPUTED,L1_FLOAT,-1.000000000,232.562332153,45.365005493,0.0,33.361850739,38.987976074,\"631T\",11,5,5,3,04,00,20,03*1f4f210e\n\tsystem status\tnormal 2 27.900000 0 0\trobot status\t166.823792\t121.906877\t7.849800\t0.136850\t-0.253794\t175.120197\t0.295000\t-0.015000\n\t\n15:43:41.0\tlog_raw\tgps_raw\t#DUALANTENNAHEADINGA,USB3,0,49.0,FINESTEERING,2107,283439.000,02000000,d426,15824;INSUFFICIENT_OBS,NONE,-1.000000000,0.000000000,0.000000000,0.0,0.000000000,0.000000000,\"631T\",12,4,4,3,04,00,20,03*4f2c0de0\n\tsystem status\tnormal 2 27.900000 0 0\trobot status\t166.678075\t121.935323\t7.849400\t0.028432\t-0.137398\t174.976327\t0.297000\t-0.009000\n\t\n15:43:41.5\tlog_raw\tgps_raw\t#DUALANTENNAHEADINGA,USB3,0,51.0,FINESTEERING,2107,283439.500,02000000,d426,15824;SOL_COMPUTED,L1_FLOAT,-1.000000000,232.643157959,45.412322998,0.0,33.247821808,38.657192230,\"631T\",11,5,5,3,04,00,20,03*dd544601\n\tsystem status\tnormal 2 27.900000 0 0\trobot status\t166.534655\t121.962304\t7.850500\t-0.095273\t-0.143173\t174.811710\t0.301000\t-0.012000\n\t\n15:43:42.0\tlog_raw\tgps_raw\t#INSPVAXA,USB3,0,51.0,FINESTEERING,2107,283440.000,02000000,471d,15824;INS_ALIGNMENT_COMPLETE,INS_RTKFIXED,37.37122940222,126.72271360028,7.8520,22.3000,0.0872,-0.2908,-0.0205,-0.014661731,-0.065843852,275.380681368,0.4409,0.2942,0.5694,0.1131,0.0924,0.0781,0.0965,0.1015,4.9875,0f000001,0*9c093e2d\n\tsystem status\tnormal 2 27.900000 0 0\trobot status\t166.394027\t121.993253\t7.852000\t-0.014662\t-0.065844\t174.619319\t0.295000\t-0.008000\n\t\n15:43:42.5\tlog_raw\tgps_raw\t#INSPVAXA,USB3,0,53.5,FINESTEERING,2107,283440.500,02000000,471d,15824;INS_ALIGNMENT_COMPLETE,INS_RTKFIXED,37.37122969334,126.72271197906,7.8553,22.3000,0.0891,-0.2848,-0.0085,0.255978109,0.004480960,275.509182296,0.4400,0.2941,0.5693,0.1129,0.0924,0.0781,0.0965,0.1015,4.9887,0f000001,0*72ef2c5e\n\tsystem status\tnormal 2 27.900000 0 0\trobot status\t166.250422\t122.025566\t7.855300\t0.255978\t0.004481\t174.490818\t0.293000\t-0.003000\n\t\n15:43:43.0\tlog_raw\tgps_raw\t#DUALANTENNAHEADINGA,USB3,0,53.5,FINESTEERING,2107,283441.000,02000000,d426,15824;INSUFFICIENT_OBS,NONE,-1.000000000,0.000000000,0.000000000,0.0,0.000000000,0.000000000,\"631T\",11,4,4,3,04,00,20,03*7d0e658d\n\tsystem status\tnormal 2 27.900000 0 0\trobot status\t166.103755\t122.059420\t7.858400\t0.290505\t-0.204110\t174.288786\t0.299000\t-0.007000\n\t\n15:43:43.5\tlog_raw\tgps_raw\t#INSPVAXA,USB3,0,48.5,FINESTEERING,2107,283441.500,02000000,471d,15824;INS_ALIGNMENT_COMPLETE,INS_RTKFIXED,37.37123027907,126.72270867931,7.8601,22.3000,0.0924,-0.3123,-0.0082,0.186564954,-0.323606469,275.889976490,0.4393,0.2940,0.5692,0.1128,0.0924,0.0781,0.0965,0.1014,4.9899,0f000001,0*5c22d510\n\tsystem status\tnormal 2 27.900000 0 0\trobot status\t165.958135\t122.090579\t7.860100\t0.186565\t-0.323606\t174.110024\t0.304000\t-0.006000\n\t\n15:43:44.0\tlog_raw\tgps_raw\t#DUALANTENNAHEADINGA,USB3,0,48.5,FINESTEERING,2107,283442.000,02000000,d426,15824;INSUFFICIENT_OBS,NONE,-1.000000000,0.000000000,0.000000000,0.0,0.000000000,0.000000000,\"631T\",12,4,4,3,04,00,20,03*81e60f26\n\tsystem status\tnormal 2 27.900000 0 0\trobot status\t165.817472\t122.124515\t7.861700\t0.206755\t-0.244335\t173.982088\t0.301000\t-0.002000\n\t\n15:43:44.5\tlog_raw\tgps_raw\t#DUALANTENNAHEADINGA,USB3,0,47.0,FINESTEERING,2107,283442.500,02000000,d426,15824;SOL_COMPUTED,L1_FLOAT,-1.000000000,232.738845825,45.537025452,0.0,33.851745605,38.946140289,\"6
